vi "websocket initialization handshake.vi"(8 "error in":errorcluster, 11 "upgrade data":T1) -> (0 "error out":errorcluster, 3 "TLS connection":refnum<class "lvlibretls connection.lvclass">)   [LabVIEW 2016, in "websocket upgrade handler.lvclass"]
uses:
  websocket upgrade handler.lvclass
  HTTP responder/http upgrade data.ctl
  lvlibtls/socket connection/lvlibretls connection.lvclass
  HTTP server/http request.ctl
  HTTP server/http method.ctl
  HTTP headers/http header data.ctl
  HTTP server/http response.ctl
  HTTP server/Basic HTTPS server.lvclass
  websocket core.lvlib
  HTTP headers/http headers.lvlib
  HTTP responder/https responder.lvclass
panel:
  out "subprotocol":string
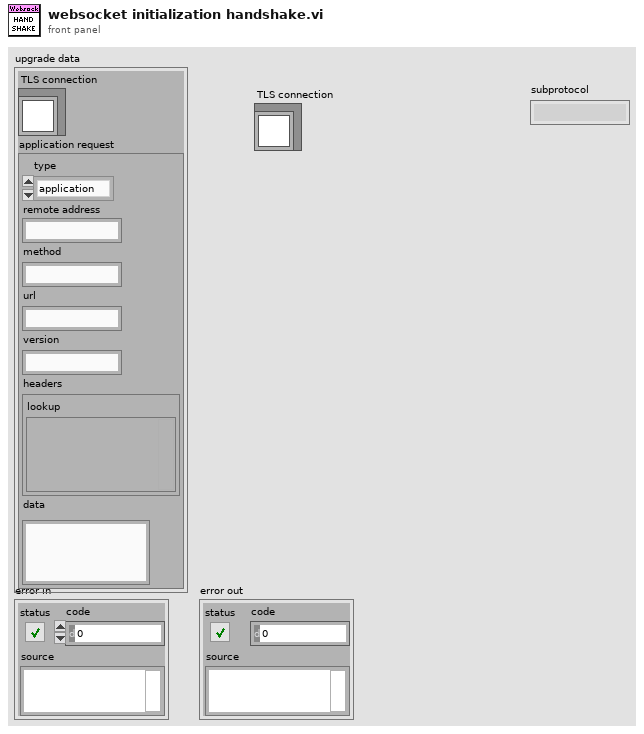
[diagram p1: front panel]
types:
  T1 = typedef "https responder.lvclass/http upgrade data.ctl" = cluster{"TLS connection":refnum<class "lvlibretls connection.lvclass">, "application request":T2}
  T2 = typedef "Basic HTTPS server.lvclass/http request.ctl" = cluster{"type":T3, "remote address":string, "method":string, "url":string, "version":string, "headers":T4, "data":string}
  T3 = typedef "Basic HTTPS server.lvclass/http method.ctl" = enum16{"application", "error", "upgrade"}
  T4 = typedef "http headers.lvlib/http header data.ctl" = cluster{"lookup":variant}
  T5 = typedef "Basic HTTPS server.lvclass/http response.ctl" = cluster{"reason code":u16, "status string":string, "headers":T4, "cookies":string[], "data":string}
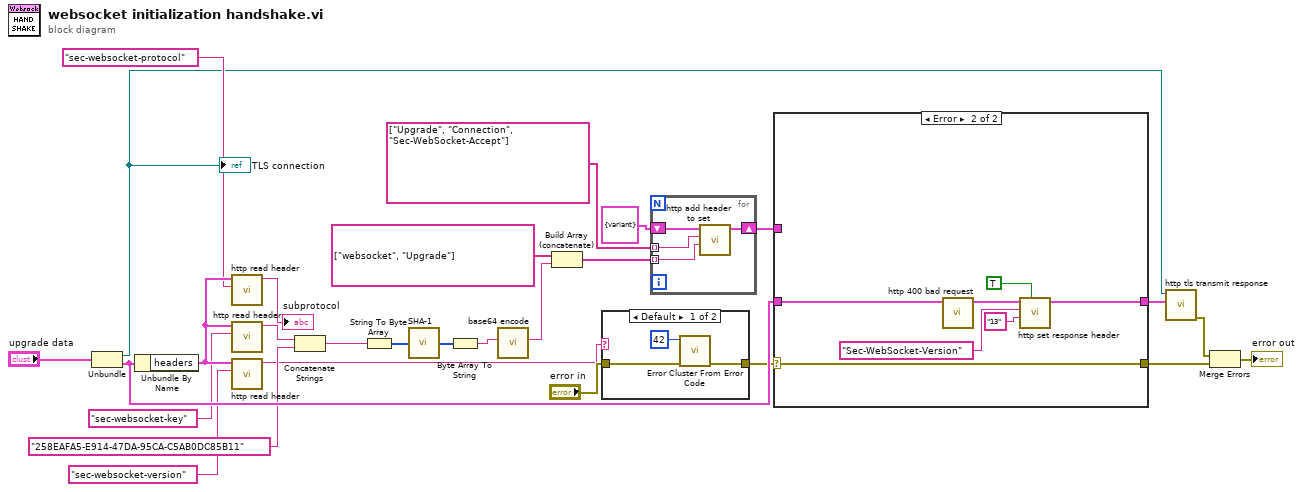
[diagram p0: block diagram]
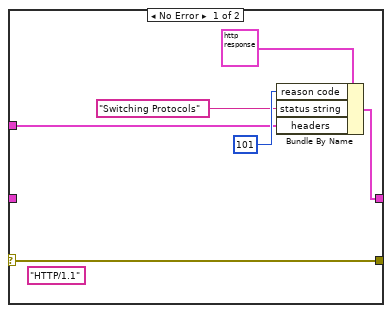
[diagram p3: hidden frame]
diagram:
  n1 = Unbundle("upgrade data") -> ("TLS connection"=w1:refnum<class "lvlibretls connection.lvclass">, "application request"=w26:T2)
  "TLS connection" <- w1
  n2 = Unbundle By Name(w26) -> ("headers"=w15:T4)
  n3 = call "http read header.vi"("header field name"="sec-websocket-protocol" ("name"), "headers"=w15) -> ("value"=→"subprotocol":string)  [unwired: 8 in, 1 out]
  n4 = call "http read header.vi"("header field name"="sec-websocket-key" ("name"), "headers"=w15) -> ("value"=w13:string)  [unwired: 8 in, 1 out]
  n5 = call "http read header.vi"("header field name"="sec-websocket-version" ("name"), "headers"=w15) -> ("value"=w11:string)  [unwired: 8 in, 1 out]
  n6 = Concatenate Strings(w13, "258EAFA5-E914-47DA-95CA-C5AB0DC85B11") -> (w21:string)
  n7 = String To Byte Array(string=w21) -> (unsigned byte array=w20:u8[])
  n8 = call "SHA-1.vi"("Data"=w20) -> ("message-digest"=w19:u8[])
  n9 = Byte Array To String(unsigned byte array=w19) -> (string=w18:string)
  n10 = call "base64 encode.vi"("string in (not encoded)"=w18) -> ("string out (base64-encoded)"=w16:string)  [unwired: 10 in]
  n11 = Build Array (concatenate)(string[] ["websocket", "Upgrade"] ("fields"), w16) -> (w4:string[])
  n12 = case shown="Default" w11 {
    tunnel: [w29 w31] -> w23
    tunnel: "error in" -> [w30 w31]
    frame Default {
      n13 = call <vilib>:"Error Cluster From Error Code.vi"("error in (no error)"=w30, "error code (0)"=42) -> ("error out"=w29:errorcluster)  [unwired: 7 in]
    }
    frame "13" {
    }
  }
  n14 = for {
    shift-right: [w32] -> w6
    shift-left: T4 {"lookup"=variant} ("headers") -> [w35]
    tunnel: string[] ["Upgrade", "Connection", "Sec-WebSocket-Accept"] ("fields") -> [w34] mode=indexing
    tunnel: w4 -> [w33] mode=indexing
    n15 = call "http add header to set.vi"("header field data"=w33, "header field name"=w34, "headers in"=w35) -> ("headers out"=w32:T4)  [unwired: 8 in]
  }
  n16 = case shown="Error" w23 {
    selector: w23 -> [w37 w47]
    tunnel: [w40 w43] -> w2
    tunnel: w26 -> [_ w48]
    tunnel: [w37 w47] -> w24
    tunnel: w6 -> [w36 _]
    frame No Error {
      (unwired) "HTTP/1.1" ("version")
      n17 = Bundle By Name(cluster=T5 {"reason code"=0, "status string"="", "headers"={"lookup"=variant}, "cookies"=[], "data"=""} ("application request"), "reason code"=u16 101, "status string"="Switching Protocols", "headers"=w36) -> (w40:T5)
    }
    frame Error {
      n18 = call "http 400 bad request.vi"("application request in"=w48) -> ("application request out"=w44:T5)  [unwired: 10 in]
      n19 = call "http set response header.vi"("override?"=TRUE, "header field data"="13" ("name"), "header field name"="Sec-WebSocket-Version" ("name"), "application request in"=w44) -> ("application request out"=w43:T5)  [unwired: 7 in]
    }
  }
  n20 = call "http tls transmit response.vi"("application request"=w2, "lvlibretls connection in"=w1) -> ("error out"=w3:errorcluster)  [unwired: 9 in]
  n21 = Merge Errors(w3, w24) -> (→"error out":errorcluster)
